vi "Delay, Seconds with Reference.vi"(4 "enable (T)":bool=TRUE, 5 "error in":errorcluster, 7 "delay":dbl[unit]=0.1 caption="Delay" format="%_3g", 8 "VISA resource":refnum<visa-resource-name>) -> (0 "error out":errorcluster {"code" format="%.0x"}, 2 "ms timer value":u32, 3 "VISA resource dup":refnum<visa-resource-name>)   [LabVIEW 2020]
doc: "Delay, if no error and enabled. For convenience, pass the VISA resource through with no modifications."
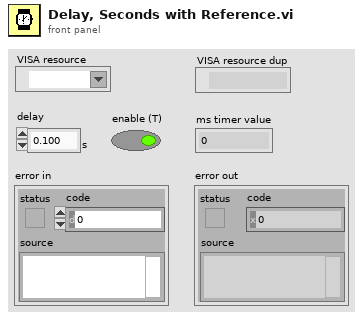
[diagram p1: front panel]
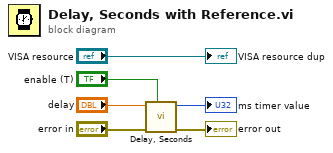
[diagram p0: block diagram]
diagram:
  n1 = call "Delay, Seconds.vi"("enable (T)"="enable (T)", "error in"="error in", "delay"="delay") -> ("error out"=→"error out":errorcluster, "ms timer value"=→"ms timer value":u32)  [unwired: 4 in]
  "VISA resource dup" <- "VISA resource"
